vi "FreqSegments.vi"(0 "VISA resource name":refnum<visa-resource-name>, 1 "FrequenciesIn":dbl[](array[numeric]), 2 "Power":dbl, 3 "error in (no error)":errorcluster, 4 "IFBW":dbl) -> (5 "VISA resource name out":refnum<visa-resource-name>, 6 "FrequenciesOut":dbl[](array[numeric]), 7 "error out":errorcluster)   [LabVIEW 2015]
uses:
  <instrlib>/Rohde&Schwarz Vector Network Analyzer/Rohde&Schwarz Vector Network Analyzer.lvlib
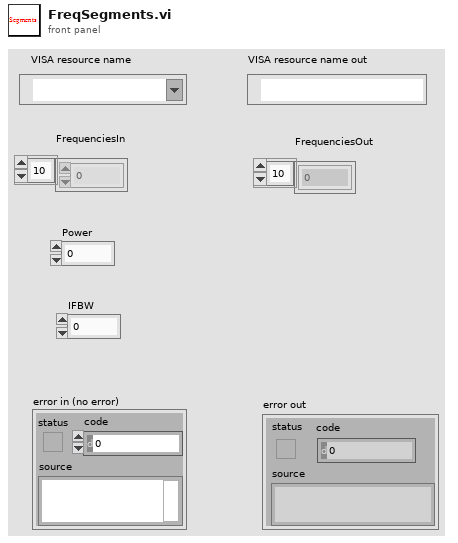
[diagram p1: front panel]
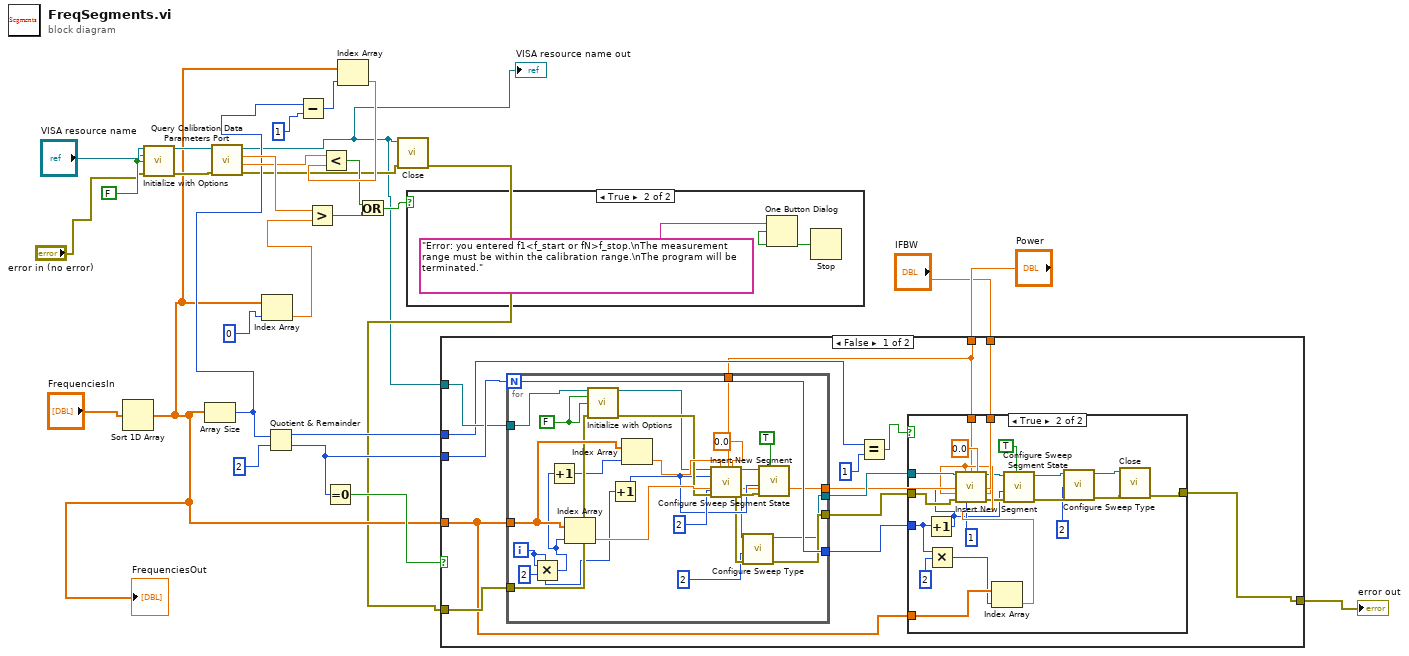
[diagram p0: block diagram]
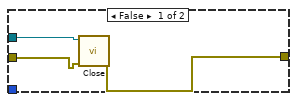
[diagram p3: hidden frame]
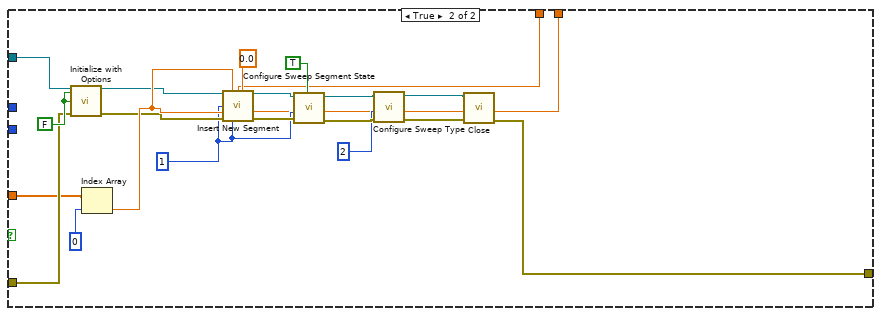
[diagram p4: hidden frame]
diagram:
  w22 = FALSE
  n1 = Sort 1D Array(array="FrequenciesIn") -> (sorted array=w10:dbl[])
  "FrequenciesOut" <- w10
  n2 = call <instrlib>:"Initialize with Options.vi"("VISA resource name"="VISA resource name", "ID Query (T: Check)"=w22, "Reset (T: Reset)"=w22, "error in (no error)"="error in (no error)") -> ("VISA resource name out"=w21:refnum<visa-resource-name>, "error out"=w20:errorcluster)  [unwired: 10 in]
  n3 = Array Size(array=w10) -> (size(s)=w13:i32)
  n4 = call <instrlib>:"Query Calibration Data Parameters Port.vi"("error in (no error)"=w20, "VISA resource name"=w21) -> ("error out"=w6:errorcluster, "Frequency Stop"=w14:dbl, "Frequency Start"=w17:dbl, "VISA resource name out"=w4:refnum<visa-resource-name>)  [unwired: 3 in, 3 out]
  "VISA resource name out" <- w4
  n5 = Index Array(array=w10, index=0) -> (element=w16:dbl)
  n6 = Quotient & Remainder(x=w13, y=2) -> (x-y*floor(x/y)=w25:i32, floor(x/y)=w26:i32)
  n7 = Subtract(x=w13, y=1) -> (x-y=w11:i32)
  n8 = Greater?(x=w17, y=w16) -> (0:w15:bool)
  n9 = Equal To 0?(x=w26) -> (x = 0?=w27:bool)
  n10 = Index Array(array=w10, index=w11) -> (element=w9:dbl)
  n11 = Less?(x=w14, y=w9) -> (x < y?=w8:bool)
  n12 = Or(x=w8, y=w15) -> (x .or. y?=w7:bool)
  n13 = call <instrlib>:"Close.vi"("error in (no error)"=w6, "VISA resource name"=w4) -> ("error out"=w5:errorcluster)  [unwired: 9 in]
  n14 = case shown="True" w7 {
    frame False {
    }
    frame True {
      n15 = One Button Dialog(message="Error: you entered f1<f_start or fN>f_stop.\nThe measurement range must be within the calibration range.\nThe program will be terminated.") -> (true=w30:bool)  [unwired: 1 in]
      n16 = Stop(stop? (T)=w30) -> ()
    }
  }
  n17 = case shown="False" w27 {
    tunnel: w4 -> [w41 w113]
    tunnel: w5 -> [w42 w112]
    tunnel: w26 -> [w43 _]
    tunnel: w25 -> [w40 _]
    tunnel: w10 -> [w34 w111]
    tunnel: [w33 w105] -> w3
    tunnel: "Power" -> [w31 w95]
    tunnel: "IFBW" -> [w32 w94]
    frame False {
      n18 = for {
        N: w43 -> [w75]
        tunnel: w34 -> [w93]
        tunnel: w42 -> [w88]
        tunnel: w41 -> [w90]
        tunnel: [w75] -> w38
        tunnel: [w73] -> w36
        tunnel: [w71] -> w35
        tunnel: w32 -> [w69]
        tunnel: w31 -> [w68]
        i -> [w80]
        w89 = FALSE
        n19 = Multiply(x=w80, y=2) -> (x*y=w82:i32)
        n20 = Increment(x=w82) -> (x+1=w81:i32)
        n21 = Index Array(array=w93, index=w82) -> (element=w92:dbl)
        n22 = call <instrlib>:"Initialize with Options.vi"("VISA resource name"=w90, "ID Query (T: Check)"=w89, "Reset (T: Reset)"=w89, "error in (no error)"=w88) -> ("VISA resource name out"=w86:refnum<visa-resource-name>, "error out"=w87:errorcluster)  [unwired: 10 in]
        n23 = Increment(x=w80) -> (x+1=w77:i32)
        n24 = Index Array(array=w93, index=w81) -> (element=w91:dbl)
        n25 = call <instrlib>:"Insert New Segment.vi"("VISA resource name"=w86, "Stop Frequency (0.0)"=w91, "Power (0.0)"=w68, "Time (21.0)"=0.0, "Segment (1)"=w77, "Start Frequency (0.0)"=w92, "Meas Bandwidth (10.0e3)"=w69, "error in (no error)"=w87, "Number Of Points (51)"=2) -> ("VISA resource name out"=w78:refnum<visa-resource-name>, "error out"=w79:errorcluster)  [unwired: 5 in]
        n26 = call <instrlib>:"Configure Sweep Segment State.vi"("State (F)"=TRUE, "error in (no error)"=w79, "Segment (1)"=w77, "VISA resource name"=w78) -> ("error out"=w74:errorcluster, "VISA resource name out"=w72:refnum<visa-resource-name>)  [unwired: 6 in]
        n27 = call <instrlib>:"Configure Sweep Type.vi"("error in (no error)"=w74, "Sweep Type (Power)"=2, "VISA resource name"=w72) -> ("error out"=w73:errorcluster, "VISA resource name out"=w71:refnum<visa-resource-name>)  [unwired: 7 in]
      }
      n28 = Equal?(x=w40, y=1) -> (x = y?=w37:bool)
      n29 = case shown="True" w37 {
        tunnel: w38 -> [_ w64]
        tunnel: w36 -> [w46 w67]
        tunnel: w35 -> [w45 w66]
        tunnel: w34 -> [_ w62]
        tunnel: [w44 w54] -> w33
        tunnel: w31 -> [_ w48]
        tunnel: w32 -> [_ w47]
        frame False {
          n30 = call <instrlib>:"Close.vi"("error in (no error)"=w46, "VISA resource name"=w45) -> ("error out"=w44:errorcluster)  [unwired: 9 in]
        }
        frame True {
          n31 = Increment(x=w64) -> (x+1=w56:i32)
          n32 = Multiply(x=w64, y=2) -> (x*y=w61:i32)
          n33 = Index Array(array=w62, index=w61) -> (element=w60:dbl)
          n34 = call <instrlib>:"Insert New Segment.vi"("VISA resource name"=w66, "Stop Frequency (0.0)"=w60, "Power (0.0)"=w48, "Time (21.0)"=0.0, "Segment (1)"=w56, "Start Frequency (0.0)"=w60, "Meas Bandwidth (10.0e3)"=w47, "error in (no error)"=w67, "Number Of Points (51)"=1) -> ("VISA resource name out"=w57:refnum<visa-resource-name>, "error out"=w58:errorcluster)  [unwired: 5 in]
          n35 = call <instrlib>:"Configure Sweep Segment State.vi"("State (F)"=TRUE, "error in (no error)"=w58, "Segment (1)"=w56, "VISA resource name"=w57) -> ("error out"=w53:errorcluster, "VISA resource name out"=w52:refnum<visa-resource-name>)  [unwired: 6 in]
          n36 = call <instrlib>:"Configure Sweep Type.vi"("error in (no error)"=w53, "Sweep Type (Power)"=2, "VISA resource name"=w52) -> ("error out"=w50:errorcluster, "VISA resource name out"=w51:refnum<visa-resource-name>)  [unwired: 7 in]
          n37 = call <instrlib>:"Close.vi"("error in (no error)"=w50, "VISA resource name"=w51) -> ("error out"=w54:errorcluster)  [unwired: 9 in]
        }
      }
    }
    frame True {
      w102 = 1
      w114 = FALSE
      n38 = call <instrlib>:"Initialize with Options.vi"("VISA resource name"=w113, "ID Query (T: Check)"=w114, "Reset (T: Reset)"=w114, "error in (no error)"=w112) -> ("VISA resource name out"=w108:refnum<visa-resource-name>, "error out"=w107:errorcluster)  [unwired: 10 in]
      n39 = Index Array(array=w111, index=0) -> (element=w109:dbl)
      n40 = call <instrlib>:"Insert New Segment.vi"("VISA resource name"=w108, "Stop Frequency (0.0)"=w109, "Power (0.0)"=w95, "Time (21.0)"=0.0, "Segment (1)"=w102, "Start Frequency (0.0)"=w109, "Meas Bandwidth (10.0e3)"=w94, "error in (no error)"=w107, "Number Of Points (51)"=w102) -> ("VISA resource name out"=w104:refnum<visa-resource-name>, "error out"=w103:errorcluster)  [unwired: 5 in]
      n41 = call <instrlib>:"Configure Sweep Segment State.vi"("State (F)"=TRUE, "error in (no error)"=w103, "Segment (1)"=w102, "VISA resource name"=w104) -> ("error out"=w100:errorcluster, "VISA resource name out"=w97:refnum<visa-resource-name>)  [unwired: 6 in]
      n42 = call <instrlib>:"Configure Sweep Type.vi"("error in (no error)"=w100, "Sweep Type (Power)"=2, "VISA resource name"=w97) -> ("error out"=w99:errorcluster, "VISA resource name out"=w98:refnum<visa-resource-name>)  [unwired: 7 in]
      n43 = call <instrlib>:"Close.vi"("error in (no error)"=w99, "VISA resource name"=w98) -> ("error out"=w105:errorcluster)  [unwired: 9 in]
    }
  }
  "error out" <- w3
